vi "ep_Search Fundamental Harmonics.vi"(7 "df":dbl format="%#_13g", 8 "error in (no error)":errorcluster, 10 "fundamental frequency [Hz]":dbl=50.0 format="%#_13g", 11 "all spectra points":cluster{"frequency":dbl[], "magnitude":dbl[]}) -> (0 "error out":errorcluster, 2 "fundamental harmonics frequencies":dbl[](array[numeric]), 3 "dup all spectra points":cluster{"frequency":dbl[], "magnitude":dbl[]})   [LabVIEW 2014, in "NI_EP_Motor Monitoring.lvlib"]
uses:
  <vilib>/addons/Electrical Power/Motor Monitoring/NI_EP_Motor Monitoring.lvlib
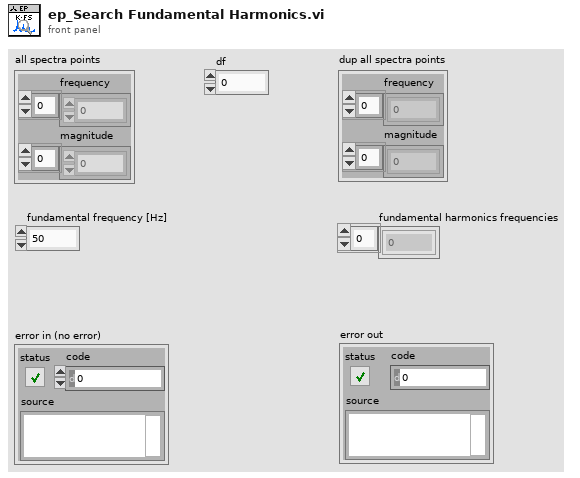
[diagram p1: front panel]
types:
  T1 = cluster{"maximum frequency [Hz]":dbl, "slip error allowance":dbl, "minimum points for peak search":dbl, "accuracy of fs":dbl, "difference?":bool, " fs harmonics order":i32, "fs forbidden range":dbl, "p3:p1 valid significance ratio":dbl, "ratio for significance weighting":dbl, "significance weighting":dbl}
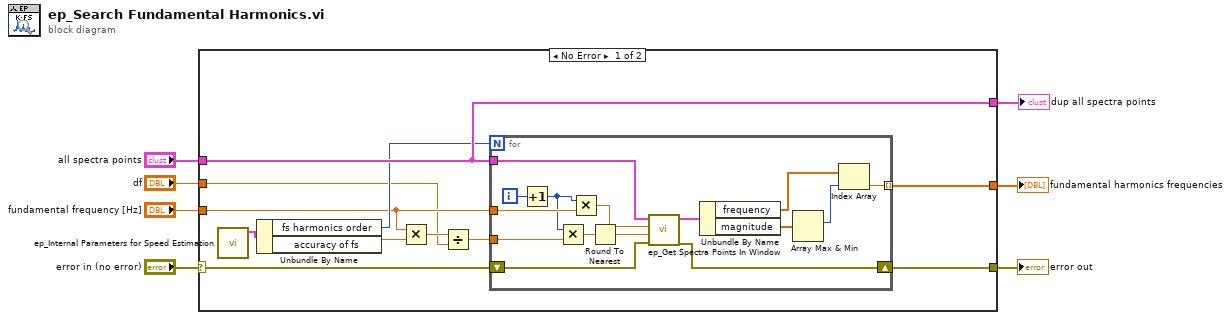
[diagram p0: block diagram]
diagram:
  n1 = case shown="No Error" "error in (no error)" {
    selector: "error in (no error)" -> [w8 w34]
    tunnel: [w18 w34] -> w6
    tunnel: "all spectra points" -> [w17 _]
    tunnel: "fundamental frequency [Hz]" -> [w11 _]
    tunnel: [w9 _] -> w3
    tunnel: [w17 _] -> w2
    tunnel: "df" -> [w10 _]
    frame No Error {
      n2 = call <vilib>:"ep_Internal Parameters for Speed Estimation.vi"() -> ("internal parameters for speed estimation"=w14:T1)  [unwired: 11 in]
      n3 = Unbundle By Name(w14) -> ("fs harmonics order"=w13:i32, "accuracy of fs"=w12:dbl)
      n4 = Multiply(x=w11, y=w12) -> (x*y=w16:dbl)
      n5 = Divide(x=w16, y=w10) -> (x/y=w15:dbl)
      n6 = for {
        N: w13 -> [_]
        tunnel: w11 -> [w33]
        tunnel: w15 -> [w22]
        tunnel: [w30] -> w9 mode=indexing
        tunnel: w17 -> [w29]
        shift-right: [w26] -> w18
        shift-left: w8 -> [w27]
        i -> [w32]
        n7 = Increment(x=w32) -> (x+1=w21:i32)
        n8 = Multiply(x=w21, y=w22) -> (x*y=w19:dbl)
        n9 = Multiply(x=w21, y=w33) -> (x*y=w28:dbl)
        n10 = Round To Nearest(number=w19) -> (nearest integer value=w20:dbl)
        n11 = call <vilib>:"ep_Get Spectra Points In Window.vi"("error in (no error)"=w27, "points of half window length"=w20, "sideband center frequency"=w28, "all spectra points"=w29) -> ("error out"=w26:errorcluster, "spectra points in window"=w25:cluster{"frequency":dbl[], "magnitude":dbl[]})  [unwired: 6 in]
        n12 = Unbundle By Name(w25) -> ("frequency"=w23:dbl[], "magnitude"=w24:dbl[])
        n13 = Array Max & Min(array=w24) -> (max index (indices)=w31:i32)  [unwired: 3 out]
        n14 = Index Array(array=w23, index=w31) -> (element=w30:dbl)
      }
    }
    frame Error {
    }
  }
  "error out" <- w6
  "fundamental harmonics frequencies" <- w3
  "dup all spectra points" <- w2
